vi "TryIncrementU8.vi"(10 "In":u8, 11 "DontInc":bool) -> (3 "Out":u8)   [LabVIEW 2018]
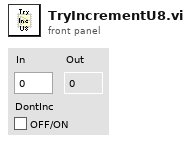
[diagram p1: front panel]
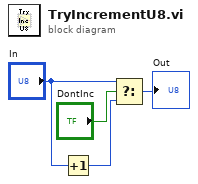
[diagram p0: block diagram]
diagram:
  n1 = Increment(x="In") -> (x+1=w3:u8)
  n2 = Select(t="In", s="DontInc", f=w3) -> (s? t:f=→"Out":u8)
